vi "Build DashBoard Data.vi"(11 "Dashboard Enables":T2={"Analog Module 1"=[TRUE, TRUE, TRUE, TRUE, TRUE, TRUE, TRUE, TRUE], "Analog Module 2"=[FALSE, FALSE, FALSE, FALSE, FALSE, FALSE, FALSE, FALSE], "Digital Module 1"=TRUE, "Digital Module 2"=FALSE, "Solenoid Module"=TRUE}) -> ()   [LabVIEW 2011]
doc: "This VI builds data and sends it back to the dashboard PC program. By default it sends back the raw values for the first analog, digital, and solenoid module. Modify it to send back the data you want to view. Consider adding higher level data to the Dashboard Datatype.ctl and to this VI. Then update the Dashboard to display the data however you like.\n\nThis software is licensed. Open the labview\\readme\\WPI Robotics Library Open Source License.txt file for more information."
uses:
  DashboardEnable.ctl
  Dashboard Datatype.ctl
  <vilib>/Rock Robotics/WPI/DriverStation/WPI_DriverStationDigitalData.ctl
  System Set Points and States.vi
panel:
  out "Dashboard Data":T1
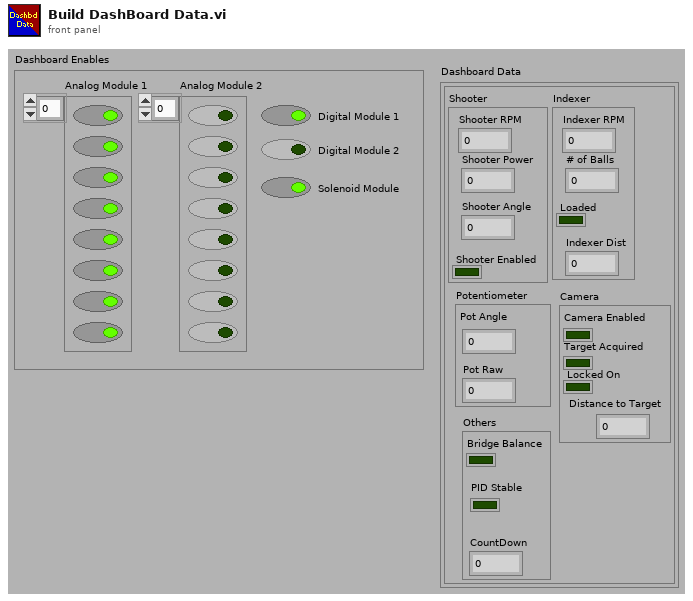
[diagram p1: front panel]
types:
  T1 = typedef "Dashboard Datatype.ctl" = cluster{"Robot Outputs":cluster{"Shooter":cluster{"Shooter RPM":dbl, "Shooter Angle":dbl, "Shooter Power":dbl, "Shooter Enabled":bool}, "Indexer":cluster{"Indexer RPM":dbl, "Loaded":bool, "# of Balls":dbl, "Indexer Dist":dbl}, "Camera":cluster{"Locked On":bool, "Target Acquired":bool, "Camera Enabled":bool, "Distance to Target":dbl}, "Potentiometer":cluster{"Pot Raw":dbl, "Pot Angle":dbl}, "Others":cluster{"CountDown":dbl, "Bridge Balance":bool, "PID Stable":bool}}}
  T2 = typedef "DashboardEnable.ctl" = cluster{"Analog Module 1":bool[], "Analog Module 2":bool[], "Digital Module 1":bool, "Digital Module 2":bool, "Solenoid Module":bool}
  T3 = typedef "WPI_DriverStationDigitalData.ctl" = cluster{"Relay Fwd":u8, "Relay Rev":u8, "GPIO":u16, "GPIO_OE":u16, "PWM":cluster{"PWM[0]":u8, "PWM[1]":u8, "PWM[2]":u8, "PWM[3]":u8, "PWM[4]":u8, "PWM[5]":u8, "PWM[6]":u8, "PWM[7]":u8, "PWM[8]":u8, "PWM[9]":u8}}
  T4 = cluster{"Shooter":cluster{"Shooter RPM":dbl, "Shooter Angle":dbl, "Shooter Power":dbl, "Shooter Enabled":bool}, "Indexer":cluster{"Indexer RPM":dbl, "Loaded":bool, "# of Balls":dbl, "Indexer Dist":dbl}, "Camera":cluster{"Locked On":bool, "Target Acquired":bool, "Camera Enabled":bool, "Distance to Target":dbl}, "Potentiometer":cluster{"Pot Raw":dbl, "Pot Angle":dbl}, "Others":cluster{"CountDown":dbl, "Bridge Balance":bool, "PID Stable":bool}}
  T5 = cluster{"Shooter RPM":dbl, "Shooter Angle":dbl, "Shooter Power":dbl, "Shooter Enabled":bool}
  T6 = cluster{"Indexer RPM":dbl, "Loaded":bool, "# of Balls":dbl, "Indexer Dist":dbl}
  T7 = cluster{"Locked On":bool, "Target Acquired":bool, "Camera Enabled":bool, "Distance to Target":dbl}
  T8 = cluster{"CountDown":dbl, "Bridge Balance":bool, "PID Stable":bool}
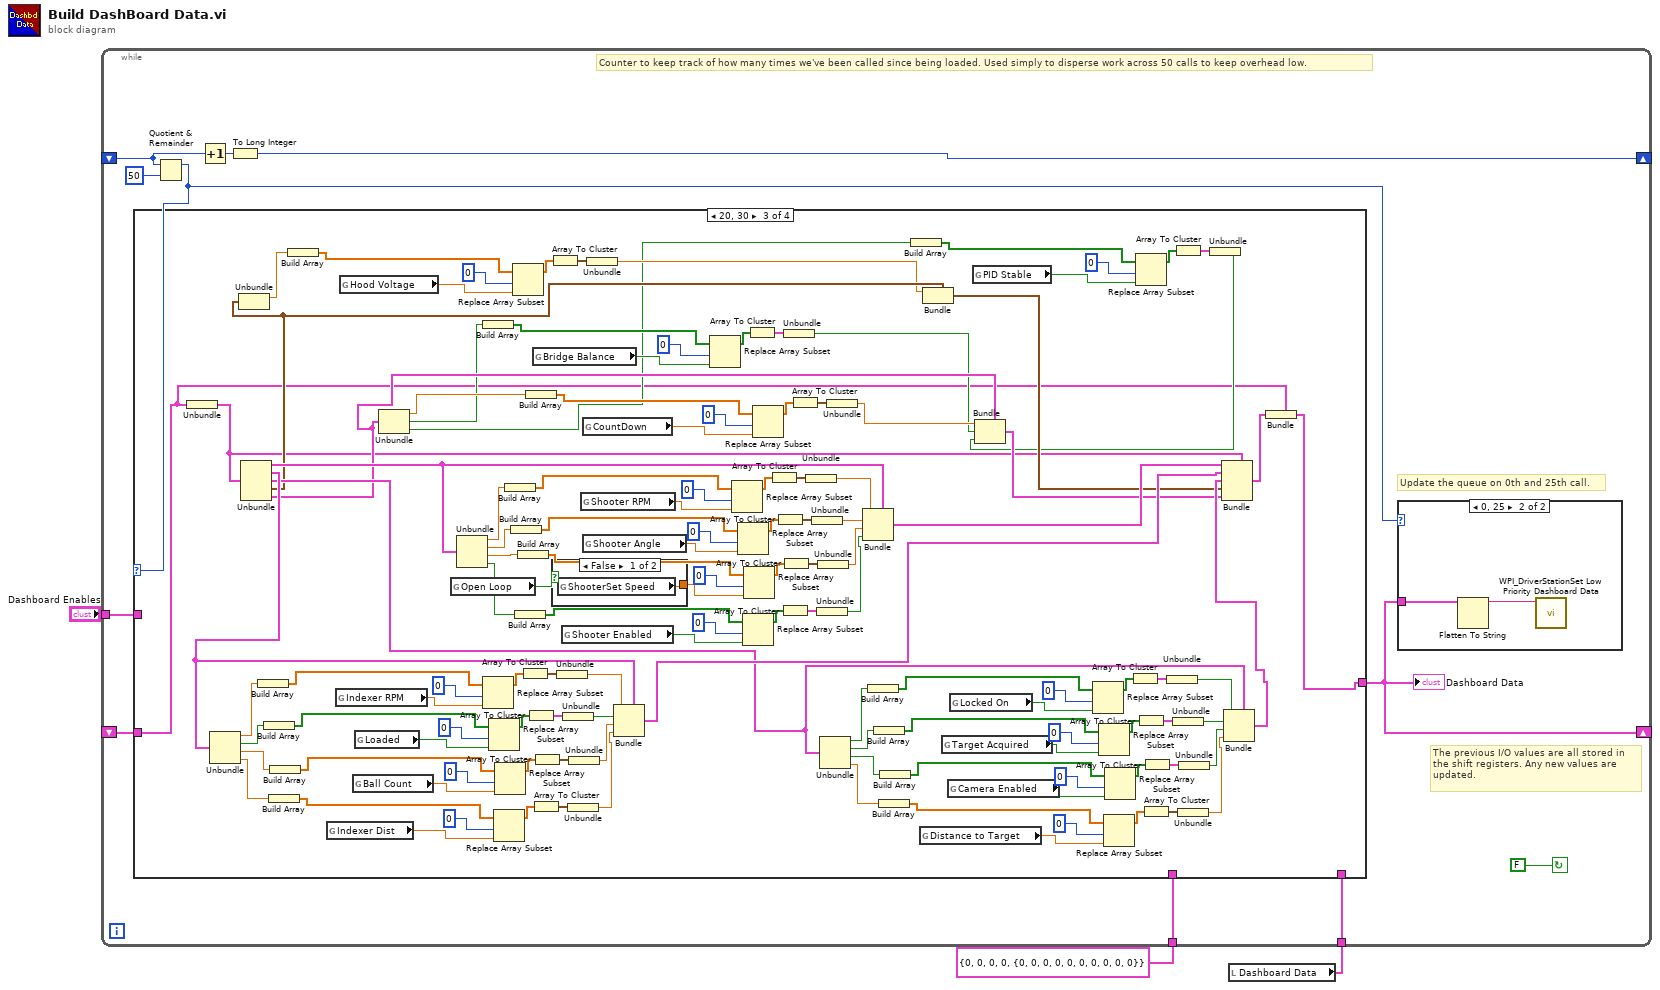
[diagram p0: block diagram]
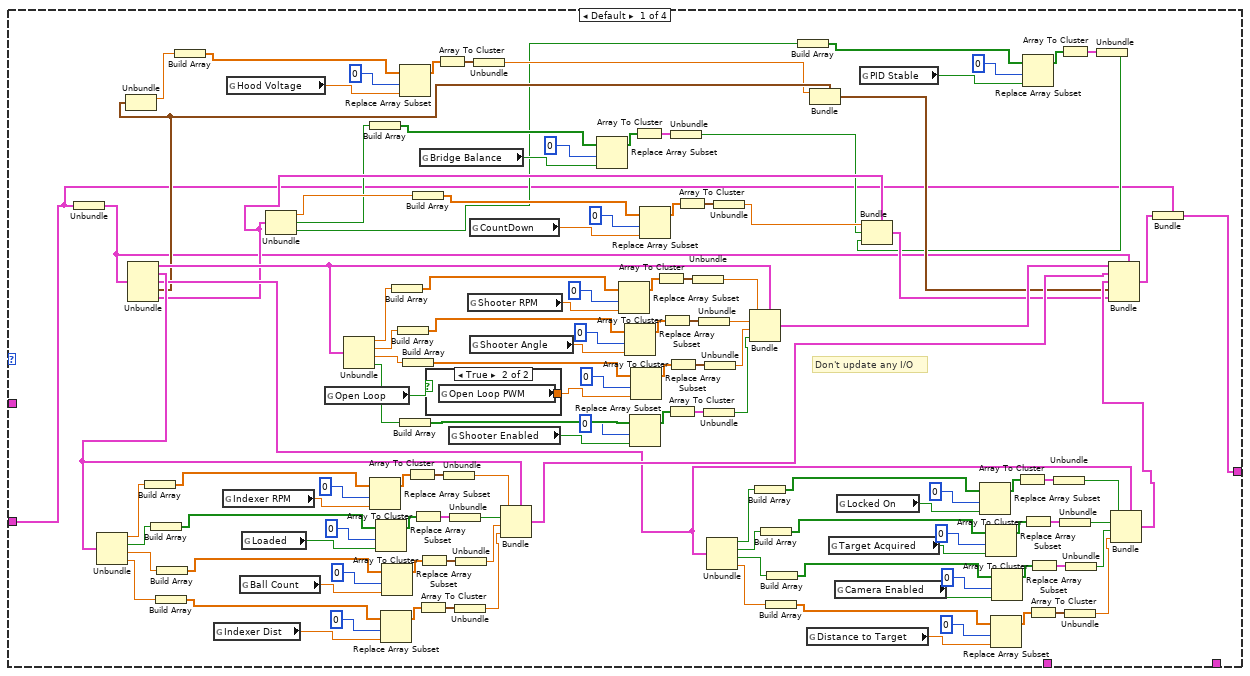
[diagram p3: hidden frame]
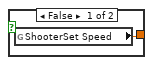
[diagram p4: hidden frame]
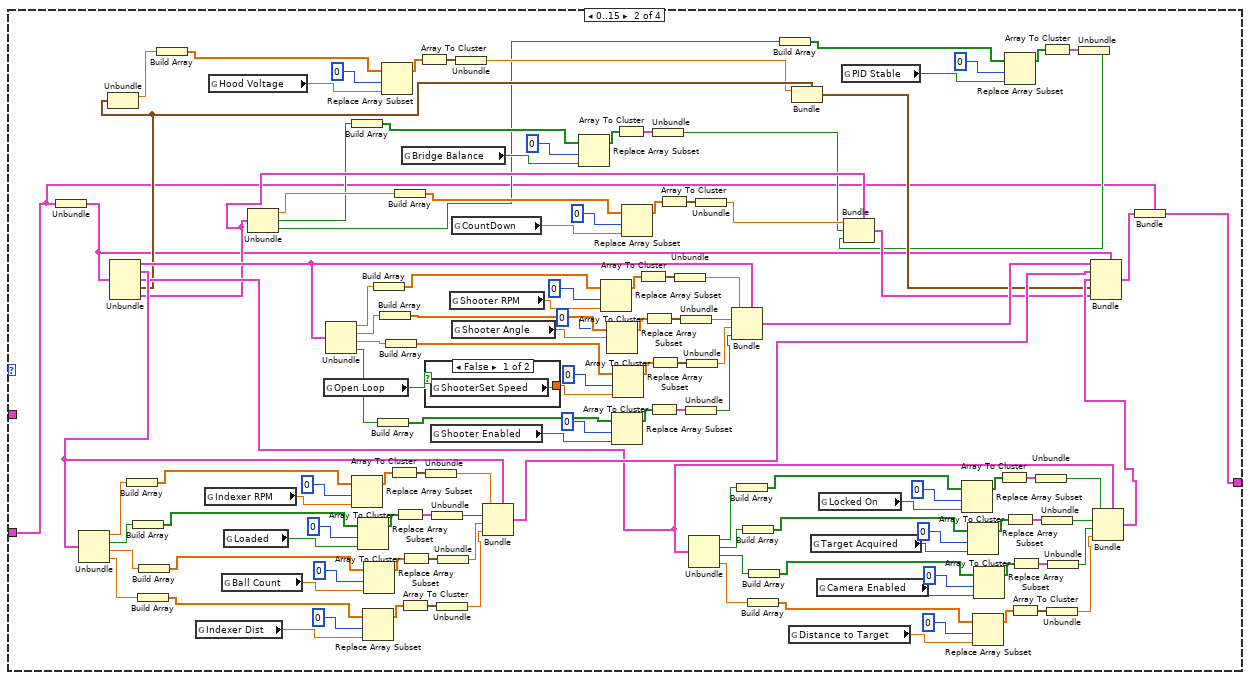
[diagram p5: hidden frame]
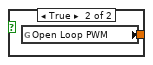
[diagram p6: hidden frame]
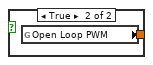
[diagram p7: hidden frame]
diagram:
  n1 = local read "Dashboard Data"() -> (w2:T1)
  n2 = while {
    shift-right: [w7] -> _
    shift-left: _ -> [w9]
    shift-right: [w4] -> _
    shift-left: _ -> [w12]
    tunnel: T3 {"Relay Fwd"=0, "Relay Rev"=0, "GPIO"=0, "GPIO_OE"=0, "PWM"={"PWM[0]"=0, "PWM[1]"=0, "PWM[2]"=0, "PWM[3]"=0, "PWM[4]"=0, "PWM[5]"=0, "PWM[6]"=0, "PWM[7]"=0, "PWM[8]"=0, "PWM[9]"=0}} ("DigitalModule[1]") -> [w11]
    tunnel: w2 -> [w6]
    tunnel: "Dashboard Enables" -> [w5]
    stop <- FALSE continue-if-true
    # "Counter to keep track of how many times we've been called since being loaded. Used simply to disperse work across 50 calls to keep overhead low."
    # "Update the queue on 0th and 25th call."
    # "The previous I/O values are all stored in\nthe shift registers. Any new values are\nupdated."
    n3 = Quotient & Remainder(x=w9, y=50) -> (x-y*floor(x/y)=w8:i32)  [unwired: 1 out]
    n4 = case shown="20, 30" w8 {
      tunnel: [w19 w150 w277 w404] -> w4
      tunnel: w12 -> [w20 w149 w278 _]
      tunnel: w11 -> [_ _ _ _]
      tunnel: w6 -> [_ _ _ w404]
      tunnel: w5 -> [_ _ _ _]
      frame Default {
        # "Don't update any I/O"
        n5 = Unbundle(w20) -> ("Robot Outputs"=w22:T4)
        n6 = Unbundle(w22) -> ("Shooter"=w142:T5, "Indexer"=w86:T6, "Camera"=w56:T7, "Potentiometer"=w33:cluster{"Pot Raw":dbl, "Pot Angle":dbl}, "Others"=w48:T8)
        n7 = Unbundle(w86) -> ("Indexer RPM"=w108:dbl, "Loaded"=w102:bool, "# of Balls"=w94:dbl, "Indexer Dist"=w88:dbl)
        n8 = Unbundle(w33) -> ("Pot Raw"=w34:dbl)  [unwired: 1 out]
        n9 = Build Array(w108) -> (w114:dbl[])
        n10 = Build Array(w102) -> (w107:bool[])
        n11 = Build Array(w88) -> (w93:dbl[])
        n12 = Build Array(w94) -> (w100:dbl[])
        n13 = Build Array(w34) -> (w39:dbl[])
        n14 = global read "System Set Points and States.vi" "Indexer Dist"() -> (w91:dbl)
        n15 = global read "System Set Points and States.vi" "Indexer RPM"() -> (w111:dbl)
        n16 = global read "System Set Points and States.vi" "Hood Voltage"() -> (w37:dbl)
        n17 = global read "System Set Points and States.vi" "Ball Count"() -> (w98:dbl)
        n18 = global read "System Set Points and States.vi" "Loaded"() -> (w105:bool)
        n19 = Unbundle(w48) -> ("CountDown"=w49:dbl, "Bridge Balance"=w41:bool, "PID Stable"=w23:bool)
        n20 = global read "System Set Points and States.vi" "Open Loop"() -> (w18:bool)
        n21 = Unbundle(w142) -> ("Shooter RPM"=w135:dbl, "Shooter Angle"=w129:dbl, "Shooter Power"=w122:dbl, "Shooter Enabled"=w116:bool)
        n22 = Build Array(w41) -> (w46:bool[])
        n23 = Replace Array Subset(array=w114, new element=w111, index=0) -> (w109:dbl[])
        n24 = Replace Array Subset(array=w107, new element=w105, index=0) -> (w103:bool[])
        n25 = Replace Array Subset(array=w93, new element=w91, index=0) -> (w89:dbl[])
        n26 = Replace Array Subset(array=w100, new element=w98, index=0) -> (w96:dbl[])
        n27 = Build Array(w135) -> (w143:dbl[])
        n28 = Build Array(w129) -> (w134:dbl[])
        n29 = Replace Array Subset(array=w39, new element=w37, index=0) -> (w35:dbl[])
        n30 = Build Array(w116) -> (w121:bool[])
        n31 = Build Array(w122) -> (w127:dbl[])
        n32 = Array To Cluster(array=w109) -> (cluster=w113:cluster{"[0]":dbl})
        n33 = Build Array(w49) -> (w54:dbl[])
        n34 = Array To Cluster(array=w103) -> (cluster=w106:cluster{"[0]":bool})
        n35 = Array To Cluster(array=w89) -> (cluster=w92:cluster{"[0]":dbl})
        n36 = Array To Cluster(array=w96) -> (cluster=w99:cluster{"[0]":dbl})
        n37 = global read "System Set Points and States.vi" "Bridge Balance"() -> (w44:bool)
        n38 = case shown="True" w18 {
          tunnel: [w144 w145] -> w17
          frame False {
            n39 = global read "System Set Points and States.vi" "ShooterSet Speed"() -> (w144:dbl)
          }
          frame True {
            n40 = global read "System Set Points and States.vi" "Open Loop PWM"() -> (w145:dbl)
          }
        }
        n41 = Array To Cluster(array=w35) -> (cluster=w38:cluster{"[0]":dbl})
        n42 = Unbundle(w113) -> ("[0]"=w112:dbl)
        n43 = global read "System Set Points and States.vi" "Shooter Enabled"() -> (w119:bool)
        n44 = Unbundle(w106) -> ("[0]"=w101:bool)
        n45 = Unbundle(w92) -> ("[0]"=w87:dbl)
        n46 = Unbundle(w99) -> ("[0]"=w95:dbl)
        n47 = global read "System Set Points and States.vi" "Shooter RPM"() -> (w138:dbl)
        n48 = global read "System Set Points and States.vi" "CountDown"() -> (w52:dbl)
        n49 = global read "System Set Points and States.vi" "Shooter Angle"() -> (w132:dbl)
        n50 = Unbundle(w38) -> ("[0]"=w32:dbl)
        n51 = Bundle(cluster=w86, "Indexer RPM"=w112, "Loaded"=w101, "# of Balls"=w95, "Indexer Dist"=w87) -> (w85:T6)
        n52 = Replace Array Subset(array=w46, new element=w44, index=0) -> (w42:bool[])
        n53 = Replace Array Subset(array=w143, new element=w138, index=0) -> (w136:dbl[])
        n54 = Replace Array Subset(array=w134, new element=w132, index=0) -> (w130:dbl[])
        n55 = Replace Array Subset(array=w121, new element=w119, index=0) -> (w117:bool[])
        n56 = Replace Array Subset(array=w127, new element=w17, index=0) -> (w124:dbl[])
        n57 = Array To Cluster(array=w42) -> (cluster=w45:cluster{"[0]":bool})
        n58 = Replace Array Subset(array=w54, new element=w52, index=0) -> (w50:dbl[])
        n59 = Array To Cluster(array=w136) -> (cluster=w141:cluster{"[0]":dbl})
        n60 = Array To Cluster(array=w130) -> (cluster=w133:cluster{"[0]":dbl})
        n61 = Array To Cluster(array=w117) -> (cluster=w120:cluster{"[0]":bool})
        n62 = Array To Cluster(array=w124) -> (cluster=w126:cluster{"[0]":dbl})
        n63 = Unbundle(w45) -> ("[0]"=w40:bool)
        n64 = Array To Cluster(array=w50) -> (cluster=w53:cluster{"[0]":dbl})
        n65 = Unbundle(w141) -> ("[0]"=w140:dbl)
        n66 = Unbundle(w133) -> ("[0]"=w128:dbl)
        n67 = Unbundle(w120) -> ("[0]"=w115:bool)
        n68 = Unbundle(w126) -> ("[0]"=w123:dbl)
        n69 = Unbundle(w56) -> ("Locked On"=w78:bool, "Target Acquired"=w72:bool, "Camera Enabled"=w64:bool, "Distance to Target"=w58:dbl)
        n70 = Unbundle(w53) -> ("[0]"=w47:dbl)
        n71 = Bundle(cluster=w142, "Shooter RPM"=w140, "Shooter Angle"=w128, "Shooter Power"=w123, "Shooter Enabled"=w115) -> (w139:T5)
        n72 = Build Array(w78) -> (w84:bool[])
        n73 = Build Array(w72) -> (w77:bool[])
        n74 = Build Array(w58) -> (w63:dbl[])
        n75 = Build Array(w64) -> (w70:bool[])
        n76 = Build Array(w23) -> (w29:bool[])
        n77 = global read "System Set Points and States.vi" "Distance to Target"() -> (w61:dbl)
        n78 = Bundle(cluster=w33, "Pot Raw"=w32) -> (w31:cluster{"Pot Raw":dbl, "Pot Angle":dbl})  [unwired: 1 in]
        n79 = global read "System Set Points and States.vi" "Target Acquired"() -> (w75:bool)
        n80 = global read "System Set Points and States.vi" "Camera Enabled"() -> (w68:bool)
        n81 = global read "System Set Points and States.vi" "Locked On"() -> (w81:bool)
        n82 = global read "System Set Points and States.vi" "PID Stable"() -> (w27:bool)
        n83 = Replace Array Subset(array=w84, new element=w81, index=0) -> (w79:bool[])
        n84 = Replace Array Subset(array=w77, new element=w75, index=0) -> (w73:bool[])
        n85 = Replace Array Subset(array=w63, new element=w61, index=0) -> (w59:dbl[])
        n86 = Replace Array Subset(array=w70, new element=w68, index=0) -> (w66:bool[])
        n87 = Array To Cluster(array=w79) -> (cluster=w83:cluster{"[0]":bool})
        n88 = Replace Array Subset(array=w29, new element=w27, index=0) -> (w25:bool[])
        n89 = Array To Cluster(array=w73) -> (cluster=w76:cluster{"[0]":bool})
        n90 = Array To Cluster(array=w59) -> (cluster=w62:cluster{"[0]":dbl})
        n91 = Array To Cluster(array=w66) -> (cluster=w69:cluster{"[0]":bool})
        n92 = Unbundle(w83) -> ("[0]"=w82:bool)
        n93 = Array To Cluster(array=w25) -> (cluster=w28:cluster{"[0]":bool})
        n94 = Unbundle(w76) -> ("[0]"=w71:bool)
        n95 = Unbundle(w62) -> ("[0]"=w57:dbl)
        n96 = Unbundle(w69) -> ("[0]"=w65:bool)
        n97 = Unbundle(w28) -> ("[0]"=w24:bool)
        n98 = Bundle(cluster=w48, "CountDown"=w47, "Bridge Balance"=w40, "PID Stable"=w24) -> (w30:T8)
        n99 = Bundle(cluster=w56, "Locked On"=w82, "Target Acquired"=w71, "Camera Enabled"=w65, "Distance to Target"=w57) -> (w55:T7)
        n100 = Bundle(cluster=w22, "Shooter"=w139, "Indexer"=w85, "Camera"=w55, "Potentiometer"=w31, "Others"=w30) -> (w21:T4)
        n101 = Bundle(cluster=w20, "Robot Outputs"=w21) -> (w19:T1)
      }
      frame 0..15 {
        n102 = Unbundle(w149) -> ("Robot Outputs"=w148:T4)
        n103 = Unbundle(w148) -> ("Shooter"=w271:T5, "Indexer"=w214:T6, "Camera"=w184:T7, "Potentiometer"=w161:cluster{"Pot Raw":dbl, "Pot Angle":dbl}, "Others"=w176:T8)
        n104 = Unbundle(w214) -> ("Indexer RPM"=w236:dbl, "Loaded"=w230:bool, "# of Balls"=w222:dbl, "Indexer Dist"=w216:dbl)
        n105 = Unbundle(w161) -> ("Pot Raw"=w162:dbl)  [unwired: 1 out]
        n106 = Build Array(w236) -> (w242:dbl[])
        n107 = Build Array(w230) -> (w235:bool[])
        n108 = Build Array(w216) -> (w221:dbl[])
        n109 = Build Array(w222) -> (w228:dbl[])
        n110 = Build Array(w162) -> (w167:dbl[])
        n111 = global read "System Set Points and States.vi" "Indexer Dist"() -> (w219:dbl)
        n112 = global read "System Set Points and States.vi" "Indexer RPM"() -> (w239:dbl)
        n113 = global read "System Set Points and States.vi" "Hood Voltage"() -> (w165:dbl)
        n114 = global read "System Set Points and States.vi" "Ball Count"() -> (w226:dbl)
        n115 = global read "System Set Points and States.vi" "Loaded"() -> (w233:bool)
        n116 = Unbundle(w176) -> ("CountDown"=w177:dbl, "Bridge Balance"=w169:bool, "PID Stable"=w151:bool)
        n117 = global read "System Set Points and States.vi" "Open Loop"() -> (w146:bool)
        n118 = Unbundle(w271) -> ("Shooter RPM"=w264:dbl, "Shooter Angle"=w258:dbl, "Shooter Power"=w250:dbl, "Shooter Enabled"=w244:bool)
        n119 = Build Array(w169) -> (w174:bool[])
        n120 = Replace Array Subset(array=w242, new element=w239, index=0) -> (w237:dbl[])
        n121 = Replace Array Subset(array=w235, new element=w233, index=0) -> (w231:bool[])
        n122 = Replace Array Subset(array=w221, new element=w219, index=0) -> (w217:dbl[])
        n123 = Replace Array Subset(array=w228, new element=w226, index=0) -> (w224:dbl[])
        n124 = Build Array(w264) -> (w272:dbl[])
        n125 = Build Array(w244) -> (w249:bool[])
        n126 = Build Array(w258) -> (w263:dbl[])
        n127 = Replace Array Subset(array=w167, new element=w165, index=0) -> (w163:dbl[])
        n128 = Build Array(w250) -> (w256:dbl[])
        n129 = Array To Cluster(array=w237) -> (cluster=w241:cluster{"[0]":dbl})
        n130 = Build Array(w177) -> (w182:dbl[])
        n131 = Array To Cluster(array=w231) -> (cluster=w234:cluster{"[0]":bool})
        n132 = Array To Cluster(array=w217) -> (cluster=w220:cluster{"[0]":dbl})
        n133 = Array To Cluster(array=w224) -> (cluster=w227:cluster{"[0]":dbl})
        n134 = global read "System Set Points and States.vi" "Bridge Balance"() -> (w172:bool)
        n135 = Array To Cluster(array=w163) -> (cluster=w166:cluster{"[0]":dbl})
        n136 = case shown="False" w146 {
          tunnel: [w273 w274] -> w254
          frame False {
            n137 = global read "System Set Points and States.vi" "ShooterSet Speed"() -> (w273:dbl)
          }
          frame True {
            n138 = global read "System Set Points and States.vi" "Open Loop PWM"() -> (w274:dbl)
          }
        }
        n139 = Unbundle(w241) -> ("[0]"=w240:dbl)
        n140 = global read "System Set Points and States.vi" "Shooter Enabled"() -> (w247:bool)
        n141 = Unbundle(w234) -> ("[0]"=w229:bool)
        n142 = Unbundle(w220) -> ("[0]"=w215:dbl)
        n143 = Unbundle(w227) -> ("[0]"=w223:dbl)
        n144 = global read "System Set Points and States.vi" "Shooter RPM"() -> (w267:dbl)
        n145 = global read "System Set Points and States.vi" "CountDown"() -> (w180:dbl)
        n146 = global read "System Set Points and States.vi" "Shooter Angle"() -> (w261:dbl)
        n147 = Unbundle(w166) -> ("[0]"=w160:dbl)
        n148 = Bundle(cluster=w214, "Indexer RPM"=w240, "Loaded"=w229, "# of Balls"=w223, "Indexer Dist"=w215) -> (w213:T6)
        n149 = Replace Array Subset(array=w174, new element=w172, index=0) -> (w170:bool[])
        n150 = Replace Array Subset(array=w272, new element=w267, index=0) -> (w265:dbl[])
        n151 = Replace Array Subset(array=w263, new element=w261, index=0) -> (w259:dbl[])
        n152 = Replace Array Subset(array=w249, new element=w247, index=0) -> (w245:bool[])
        n153 = Replace Array Subset(array=w256, new element=w254, index=0) -> (w252:dbl[])
        n154 = Array To Cluster(array=w170) -> (cluster=w173:cluster{"[0]":bool})
        n155 = Replace Array Subset(array=w182, new element=w180, index=0) -> (w178:dbl[])
        n156 = Array To Cluster(array=w265) -> (cluster=w270:cluster{"[0]":dbl})
        n157 = Array To Cluster(array=w259) -> (cluster=w262:cluster{"[0]":dbl})
        n158 = Array To Cluster(array=w245) -> (cluster=w248:cluster{"[0]":bool})
        n159 = Array To Cluster(array=w252) -> (cluster=w255:cluster{"[0]":dbl})
        n160 = Unbundle(w173) -> ("[0]"=w168:bool)
        n161 = Array To Cluster(array=w178) -> (cluster=w181:cluster{"[0]":dbl})
        n162 = Unbundle(w270) -> ("[0]"=w269:dbl)
        n163 = Unbundle(w262) -> ("[0]"=w257:dbl)
        n164 = Unbundle(w248) -> ("[0]"=w243:bool)
        n165 = Unbundle(w255) -> ("[0]"=w251:dbl)
        n166 = Unbundle(w184) -> ("Locked On"=w206:bool, "Target Acquired"=w200:bool, "Camera Enabled"=w192:bool, "Distance to Target"=w186:dbl)
        n167 = Unbundle(w181) -> ("[0]"=w175:dbl)
        n168 = Bundle(cluster=w271, "Shooter RPM"=w269, "Shooter Angle"=w257, "Shooter Power"=w251, "Shooter Enabled"=w243) -> (w268:T5)
        n169 = Build Array(w206) -> (w212:bool[])
        n170 = Build Array(w200) -> (w205:bool[])
        n171 = Build Array(w186) -> (w191:dbl[])
        n172 = Build Array(w192) -> (w198:bool[])
        n173 = Build Array(w151) -> (w157:bool[])
        n174 = global read "System Set Points and States.vi" "Distance to Target"() -> (w189:dbl)
        n175 = Bundle(cluster=w161, "Pot Raw"=w160) -> (w159:cluster{"Pot Raw":dbl, "Pot Angle":dbl})  [unwired: 1 in]
        n176 = global read "System Set Points and States.vi" "Target Acquired"() -> (w203:bool)
        n177 = global read "System Set Points and States.vi" "Camera Enabled"() -> (w196:bool)
        n178 = global read "System Set Points and States.vi" "Locked On"() -> (w209:bool)
        n179 = global read "System Set Points and States.vi" "PID Stable"() -> (w155:bool)
        n180 = Replace Array Subset(array=w212, new element=w209, index=0) -> (w207:bool[])
        n181 = Replace Array Subset(array=w205, new element=w203, index=0) -> (w201:bool[])
        n182 = Replace Array Subset(array=w191, new element=w189, index=0) -> (w187:dbl[])
        n183 = Replace Array Subset(array=w198, new element=w196, index=0) -> (w194:bool[])
        n184 = Array To Cluster(array=w207) -> (cluster=w211:cluster{"[0]":bool})
        n185 = Replace Array Subset(array=w157, new element=w155, index=0) -> (w153:bool[])
        n186 = Array To Cluster(array=w201) -> (cluster=w204:cluster{"[0]":bool})
        n187 = Array To Cluster(array=w187) -> (cluster=w190:cluster{"[0]":dbl})
        n188 = Array To Cluster(array=w194) -> (cluster=w197:cluster{"[0]":bool})
        n189 = Unbundle(w211) -> ("[0]"=w210:bool)
        n190 = Array To Cluster(array=w153) -> (cluster=w156:cluster{"[0]":bool})
        n191 = Unbundle(w204) -> ("[0]"=w199:bool)
        n192 = Unbundle(w190) -> ("[0]"=w185:dbl)
        n193 = Unbundle(w197) -> ("[0]"=w193:bool)
        n194 = Unbundle(w156) -> ("[0]"=w152:bool)
        n195 = Bundle(cluster=w176, "CountDown"=w175, "Bridge Balance"=w168, "PID Stable"=w152) -> (w158:T8)
        n196 = Bundle(cluster=w184, "Locked On"=w210, "Target Acquired"=w199, "Camera Enabled"=w193, "Distance to Target"=w185) -> (w183:T7)
        n197 = Bundle(cluster=w148, "Shooter"=w268, "Indexer"=w213, "Camera"=w183, "Potentiometer"=w159, "Others"=w158) -> (w147:T4)
        n198 = Bundle(cluster=w149, "Robot Outputs"=w147) -> (w150:T1)
      }
      frame 20, 30 {
        n199 = Unbundle(w278) -> ("Robot Outputs"=w280:T4)
        n200 = Unbundle(w280) -> ("Shooter"=w400:T5, "Indexer"=w344:T6, "Camera"=w314:T7, "Potentiometer"=w291:cluster{"Pot Raw":dbl, "Pot Angle":dbl}, "Others"=w306:T8)
        n201 = Unbundle(w344) -> ("Indexer RPM"=w366:dbl, "Loaded"=w360:bool, "# of Balls"=w352:dbl, "Indexer Dist"=w346:dbl)
        n202 = Unbundle(w291) -> ("Pot Raw"=w292:dbl)  [unwired: 1 out]
        n203 = Build Array(w366) -> (w372:dbl[])
        n204 = Build Array(w360) -> (w365:bool[])
        n205 = Build Array(w346) -> (w351:dbl[])
        n206 = Build Array(w352) -> (w358:dbl[])
        n207 = Build Array(w292) -> (w297:dbl[])
        n208 = global read "System Set Points and States.vi" "Indexer Dist"() -> (w349:dbl)
        n209 = global read "System Set Points and States.vi" "Indexer RPM"() -> (w369:dbl)
        n210 = global read "System Set Points and States.vi" "Hood Voltage"() -> (w295:dbl)
        n211 = global read "System Set Points and States.vi" "Ball Count"() -> (w356:dbl)
        n212 = global read "System Set Points and States.vi" "Loaded"() -> (w363:bool)
        n213 = Unbundle(w306) -> ("CountDown"=w307:dbl, "Bridge Balance"=w299:bool, "PID Stable"=w281:bool)
        n214 = global read "System Set Points and States.vi" "Open Loop"() -> (w276:bool)
        n215 = Unbundle(w400) -> ("Shooter RPM"=w393:dbl, "Shooter Angle"=w387:dbl, "Shooter Power"=w380:dbl, "Shooter Enabled"=w374:bool)
        n216 = Build Array(w299) -> (w304:bool[])
        n217 = Replace Array Subset(array=w372, new element=w369, index=0) -> (w367:dbl[])
        n218 = Replace Array Subset(array=w365, new element=w363, index=0) -> (w361:bool[])
        n219 = Replace Array Subset(array=w351, new element=w349, index=0) -> (w347:dbl[])
        n220 = Replace Array Subset(array=w358, new element=w356, index=0) -> (w354:dbl[])
        n221 = Build Array(w393) -> (w401:dbl[])
        n222 = Build Array(w387) -> (w392:dbl[])
        n223 = Replace Array Subset(array=w297, new element=w295, index=0) -> (w293:dbl[])
        n224 = Build Array(w374) -> (w379:bool[])
        n225 = Build Array(w380) -> (w385:dbl[])
        n226 = Array To Cluster(array=w367) -> (cluster=w371:cluster{"[0]":dbl})
        n227 = Build Array(w307) -> (w312:dbl[])
        n228 = Array To Cluster(array=w361) -> (cluster=w364:cluster{"[0]":bool})
        n229 = Array To Cluster(array=w347) -> (cluster=w350:cluster{"[0]":dbl})
        n230 = Array To Cluster(array=w354) -> (cluster=w357:cluster{"[0]":dbl})
        n231 = global read "System Set Points and States.vi" "Bridge Balance"() -> (w302:bool)
        n232 = Array To Cluster(array=w293) -> (cluster=w296:cluster{"[0]":dbl})
        n233 = case shown="False" w276 {
          tunnel: [w402 w403] -> w275
          frame False {
            n234 = global read "System Set Points and States.vi" "ShooterSet Speed"() -> (w402:dbl)
          }
          frame True {
            n235 = global read "System Set Points and States.vi" "Open Loop PWM"() -> (w403:dbl)
          }
        }
        n236 = Unbundle(w371) -> ("[0]"=w370:dbl)
        n237 = global read "System Set Points and States.vi" "Shooter Enabled"() -> (w377:bool)
        n238 = Unbundle(w364) -> ("[0]"=w359:bool)
        n239 = Unbundle(w350) -> ("[0]"=w345:dbl)
        n240 = Unbundle(w357) -> ("[0]"=w353:dbl)
        n241 = global read "System Set Points and States.vi" "Shooter RPM"() -> (w396:dbl)
        n242 = global read "System Set Points and States.vi" "CountDown"() -> (w310:dbl)
        n243 = global read "System Set Points and States.vi" "Shooter Angle"() -> (w390:dbl)
        n244 = Unbundle(w296) -> ("[0]"=w290:dbl)
        n245 = Bundle(cluster=w344, "Indexer RPM"=w370, "Loaded"=w359, "# of Balls"=w353, "Indexer Dist"=w345) -> (w343:T6)
        n246 = Replace Array Subset(array=w304, new element=w302, index=0) -> (w300:bool[])
        n247 = Replace Array Subset(array=w401, new element=w396, index=0) -> (w394:dbl[])
        n248 = Replace Array Subset(array=w392, new element=w390, index=0) -> (w388:dbl[])
        n249 = Replace Array Subset(array=w379, new element=w377, index=0) -> (w375:bool[])
        n250 = Replace Array Subset(array=w385, new element=w275, index=0) -> (w382:dbl[])
        n251 = Array To Cluster(array=w300) -> (cluster=w303:cluster{"[0]":bool})
        n252 = Replace Array Subset(array=w312, new element=w310, index=0) -> (w308:dbl[])
        n253 = Array To Cluster(array=w394) -> (cluster=w399:cluster{"[0]":dbl})
        n254 = Array To Cluster(array=w388) -> (cluster=w391:cluster{"[0]":dbl})
        n255 = Array To Cluster(array=w375) -> (cluster=w378:cluster{"[0]":bool})
        n256 = Array To Cluster(array=w382) -> (cluster=w384:cluster{"[0]":dbl})
        n257 = Unbundle(w303) -> ("[0]"=w298:bool)
        n258 = Array To Cluster(array=w308) -> (cluster=w311:cluster{"[0]":dbl})
        n259 = Unbundle(w399) -> ("[0]"=w398:dbl)
        n260 = Unbundle(w391) -> ("[0]"=w386:dbl)
        n261 = Unbundle(w378) -> ("[0]"=w373:bool)
        n262 = Unbundle(w384) -> ("[0]"=w381:dbl)
        n263 = Unbundle(w314) -> ("Locked On"=w336:bool, "Target Acquired"=w330:bool, "Camera Enabled"=w322:bool, "Distance to Target"=w316:dbl)
        n264 = Unbundle(w311) -> ("[0]"=w305:dbl)
        n265 = Bundle(cluster=w400, "Shooter RPM"=w398, "Shooter Angle"=w386, "Shooter Power"=w381, "Shooter Enabled"=w373) -> (w397:T5)
        n266 = Build Array(w336) -> (w342:bool[])
        n267 = Build Array(w330) -> (w335:bool[])
        n268 = Build Array(w316) -> (w321:dbl[])
        n269 = Build Array(w322) -> (w328:bool[])
        n270 = Build Array(w281) -> (w287:bool[])
        n271 = global read "System Set Points and States.vi" "Distance to Target"() -> (w319:dbl)
        n272 = Bundle(cluster=w291, "Pot Raw"=w290) -> (w289:cluster{"Pot Raw":dbl, "Pot Angle":dbl})  [unwired: 1 in]
        n273 = global read "System Set Points and States.vi" "Target Acquired"() -> (w333:bool)
        n274 = global read "System Set Points and States.vi" "Camera Enabled"() -> (w326:bool)
        n275 = global read "System Set Points and States.vi" "Locked On"() -> (w339:bool)
        n276 = global read "System Set Points and States.vi" "PID Stable"() -> (w285:bool)
        n277 = Replace Array Subset(array=w342, new element=w339, index=0) -> (w337:bool[])
        n278 = Replace Array Subset(array=w335, new element=w333, index=0) -> (w331:bool[])
        n279 = Replace Array Subset(array=w321, new element=w319, index=0) -> (w317:dbl[])
        n280 = Replace Array Subset(array=w328, new element=w326, index=0) -> (w324:bool[])
        n281 = Array To Cluster(array=w337) -> (cluster=w341:cluster{"[0]":bool})
        n282 = Replace Array Subset(array=w287, new element=w285, index=0) -> (w283:bool[])
        n283 = Array To Cluster(array=w331) -> (cluster=w334:cluster{"[0]":bool})
        n284 = Array To Cluster(array=w317) -> (cluster=w320:cluster{"[0]":dbl})
        n285 = Array To Cluster(array=w324) -> (cluster=w327:cluster{"[0]":bool})
        n286 = Unbundle(w341) -> ("[0]"=w340:bool)
        n287 = Array To Cluster(array=w283) -> (cluster=w286:cluster{"[0]":bool})
        n288 = Unbundle(w334) -> ("[0]"=w329:bool)
        n289 = Unbundle(w320) -> ("[0]"=w315:dbl)
        n290 = Unbundle(w327) -> ("[0]"=w323:bool)
        n291 = Unbundle(w286) -> ("[0]"=w282:bool)
        n292 = Bundle(cluster=w306, "CountDown"=w305, "Bridge Balance"=w298, "PID Stable"=w282) -> (w288:T8)
        n293 = Bundle(cluster=w314, "Locked On"=w340, "Target Acquired"=w329, "Camera Enabled"=w323, "Distance to Target"=w315) -> (w313:T7)
        n294 = Bundle(cluster=w280, "Shooter"=w397, "Indexer"=w343, "Camera"=w313, "Potentiometer"=w289, "Others"=w288) -> (w279:T4)
        n295 = Bundle(cluster=w278, "Robot Outputs"=w279) -> (w277:T1)
      }
      frame 40 {
      }
    }
    "Dashboard Data" <- w4
    n296 = Increment(x=w9) -> (x+1=w14:i32)
    n297 = To Long Integer(number=w14) -> (32bit integer=w7:i32)
    n298 = case shown="0, 25" w8 {
      tunnel: w4 -> [_ w16]
      frame Default {
      }
      frame 0, 25 {
        n299 = Flatten To String(anything=w16) -> (data string=w15:string)  [unwired: 1 in, 4 out]
        n300 = call <vilib>:"WPI_DriverStationSet Low Priority Dashboard Data.vi"("User Data"=w15) -> ()  [unwired: 1 in, 10 out]
      }
    }
  }
